vi "Signal Checker.vi"(3 "error in":errorcluster, 4 "Task to Check Array":refnum<k21>[](array[refnum]), 5 "milliseconds to wait":u32) -> (0 "error out":errorcluster, 2 "Warning Num":i32)   [LabVIEW 2013]
uses:
  <vilib>/DAQmx/read.llb/DAQmx Read (Digital 1D Bool NChan 1Samp 1Line).vi
  <vilib>/DAQmx/miscellaneous.llb/DAQmx Fill In Error Info.vi
panel:
  out "Text.Text":string
  out "P0L0 out Array 3":refnum<k21>[](array[refnum])
  out "element":refnum<k21>
  out "P0L0 out Array 2":refnum<k21>[](array[refnum])
  out "P0L0 out Array":refnum<k21>[](array[refnum])
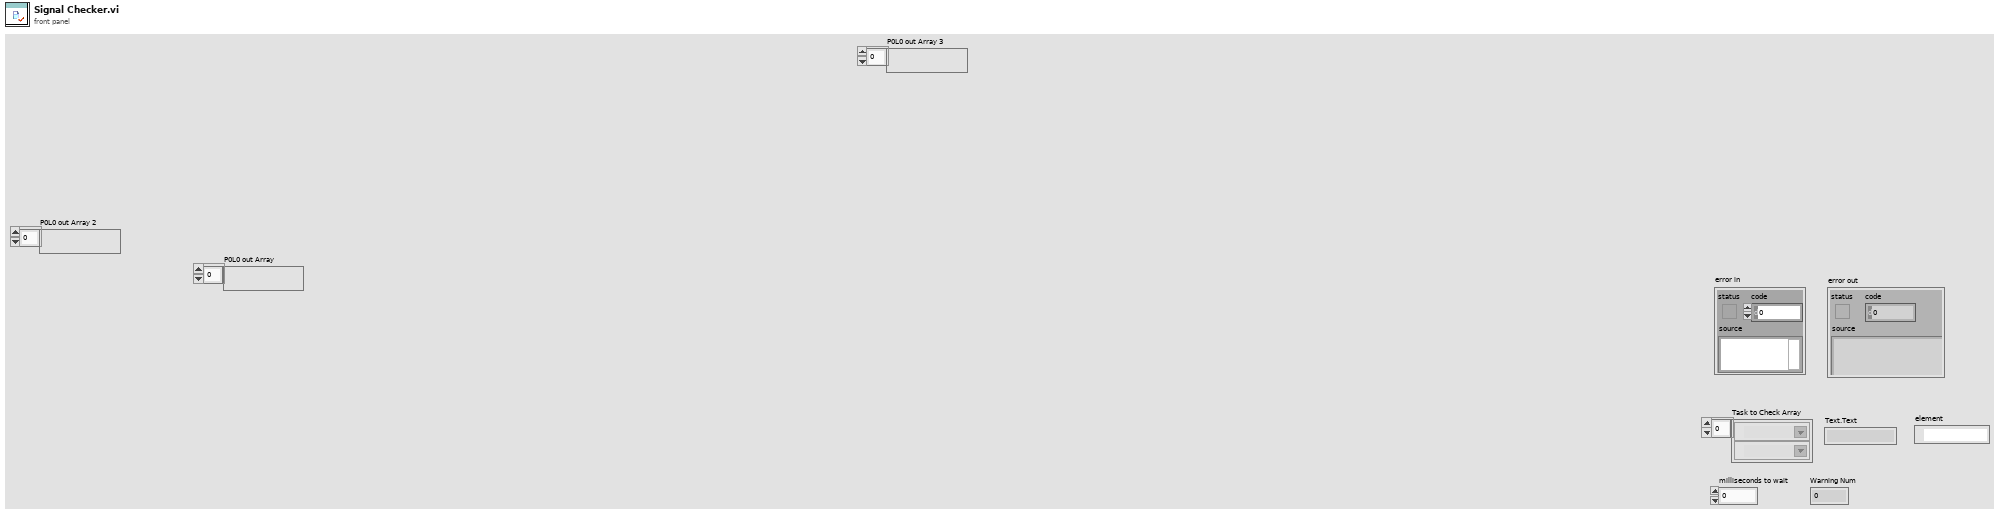
[diagram p1: front panel]
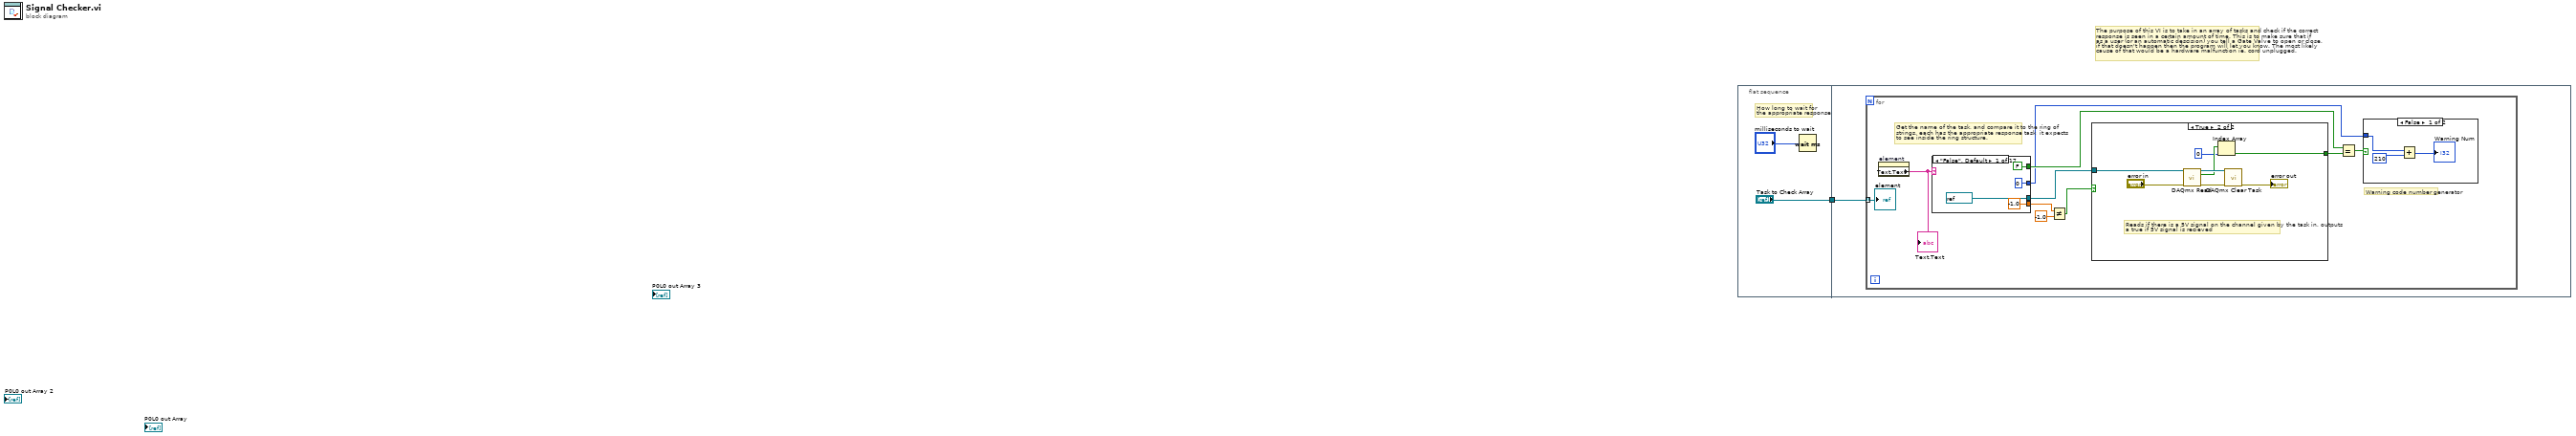
[diagram p0: block diagram]
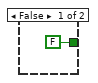
[diagram p3: hidden frame]
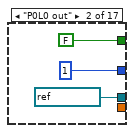
[diagram p4: hidden frame]
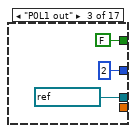
[diagram p5: hidden frame]
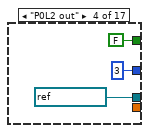
[diagram p6: hidden frame]
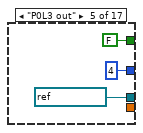
[diagram p7: hidden frame]
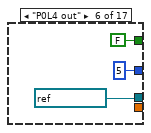
[diagram p8: hidden frame]
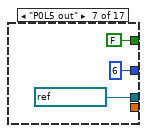
[diagram p9: hidden frame]
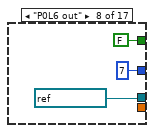
[diagram p10: hidden frame]
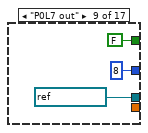
[diagram p11: hidden frame]
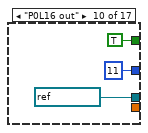
[diagram p12: hidden frame]
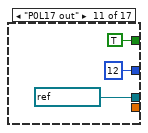
[diagram p13: hidden frame]
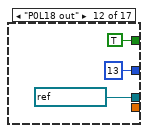
[diagram p14: hidden frame]
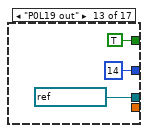
[diagram p15: hidden frame]
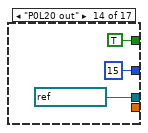
[diagram p16: hidden frame]
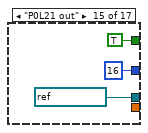
[diagram p17: hidden frame]
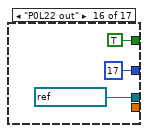
[diagram p18: hidden frame]
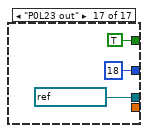
[diagram p19: hidden frame]
diagram:
  # "The purpose of this VI is to take in an array of tasks and check if the correct\nresponse is seen in a certain amount of time. This is to make sure that if \nas a user (or an automatic descision) you tell a Gate Valve to open or close,\nif that doesn't happen then the program will let you know. The most likely \ncause of that would be a hardware malfunction ie. cord unplugged."
  n1 = flat-sequence {
    tunnel: ["Task to Check Array"] -> w1
    tunnel: w1 -> [w4]
    frame #0 {
      # "How long to wait for \nthe appropriate response"
      n2 = Wait (ms)(milliseconds to wait="milliseconds to wait") -> ()  [unwired: 1 out]
    }
    frame #1 {
      n3 = for {
        tunnel: w4 -> [w8] mode=indexing
        # "Warning code number generator"
        # "Get the name of the task, and compare it to the ring of\nstrings, each has the appropriate response task  it expects\nto see inside the ring structure."
        n4 = property on="element" class="DAQmxName (strict)"() -> ("Text.Text"=w14:string)  [unwired: 2 in, 2 out]
        "Text.Text" <- w14
        n5 = case shown="\"False\", Default" w14 {
          tunnel: [refnum<k21> "test" ("DAQmx Task Name") refnum<k21> "P0L8 in" ("DAQmx Task Name") refnum<k21> "P0L9 in" ("DAQmx Task Name") refnum<k21> "P0L10 in" ("DAQmx Task Name") refnum<k21> "P0L11 in" ("DAQmx Task Name") refnum<k21> "P0L12 in" ("DAQmx Task Name") refnum<k21> "P0L13 in" ("DAQmx Task Name") refnum<k21> "P0L14 in" ("DAQmx Task Name") refnum<k21> "P0L15 in" ("DAQmx Task Name") refnum<k21> "P0L8 in" ("DAQmx Task Name") refnum<k21> "P0L9 in" ("DAQmx Task Name") refnum<k21> "P0L10 in" ("DAQmx Task Name") refnum<k21> "P0L11 in" ("DAQmx Task Name") refnum<k21> "P0L12 in" ("DAQmx Task Name") refnum<k21> "P0L13 in" ("DAQmx Task Name") refnum<k21> "P0L14 in" ("DAQmx Task Name") refnum<k21> "P0L15 in" ("DAQmx Task Name")] -> w13
          tunnel: [FALSE FALSE FALSE FALSE FALSE FALSE FALSE FALSE FALSE TRUE TRUE TRUE TRUE TRUE TRUE TRUE TRUE] -> w10
          tunnel: [-1.0 ("y") _ _ _ _ _ _ _ _ _ _ _ _ _ _ _ _] -> w6
          tunnel: [0 1 2 3 4 5 6 7 8 11 12 13 14 15 16 17 18] -> w5
          frame "False", Default {
          }
          frame "P0L0 out" {
          }
          frame "P0L1 out" {
          }
          frame "P0L2 out" {
          }
          frame "P0L3 out" {
          }
          frame "P0L4 out" {
          }
          frame "P0L5 out" {
          }
          frame "P0L6 out" {
          }
          frame "P0L7 out" {
          }
          frame "P0L16 out" {
          }
          frame "P0L17 out" {
          }
          frame "P0L18 out" {
          }
          frame "P0L19 out" {
          }
          frame "P0L20 out" {
          }
          frame "P0L21 out" {
          }
          frame "P0L22 out" {
          }
          frame "P0L23 out" {
          }
        }
        n6 = Not Equal?(x=w6, y=-1.0) -> (x != y?=w12:bool)
        n7 = case shown="True" w12 {
          tunnel: [FALSE ("Boolean") w20] -> w11
          tunnel: w13 -> [_ w19]
          frame False {
          }
          frame True {
            # "Reads if there is a 5V signal on the channel given by the task in, outputs\na true if 5V signal is recieved"
            n8 = call-poly <vilib>:"DAQmx Read.vi"("task/channels in"=w19, "error in"="error in") -> ("task out"=w25:refnum<k21>, "data"=w23:bool[], "error out"=w26:errorcluster)  [unwired: 11 in]
            n9 = Index Array(array=w23, index=0) -> (element=w20:bool)
            n10 = call <vilib>:"DAQmx Clear Task.vi"("task in"=w25, "error in"=w26) -> ("error out"=→"error out":errorcluster)  [unwired: 13 in]
          }
        }
        n11 = Equal?(x=w10, y=w11) -> (x = y?=w9:bool)
        n12 = case shown="False" w9 {
          tunnel: w5 -> [w17 _]
          frame False {
            n13 = Add(x=w17, y=210) -> (x+y=→"Warning Num":i32)
          }
          frame True {
          }
        }
        "element" <- w8
      }
    }
  }
